vi "Picolog Close Device.vi"(8 "Error In":errorcluster, 11 "Instrument Handle":i16=1) -> (0 "Error Out":errorcluster)   [LabVIEW 2017]
uses:
  usbtc08.dll
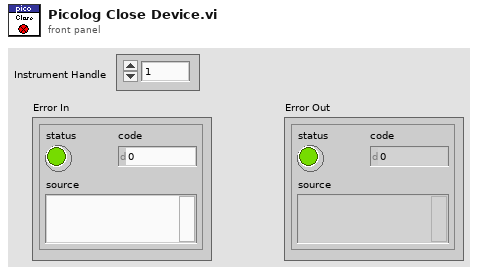
[diagram p1: front panel]
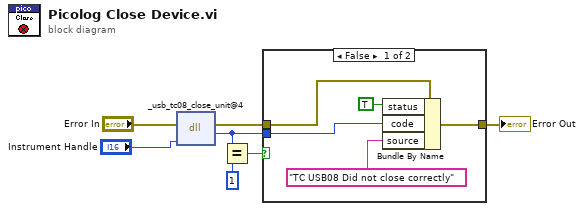
[diagram p0: block diagram]
diagram:
  n1 = dll-call lib="usbtc08.dll" fn="_usb_tc08_close_unit@4" label="Close unit"(error in="Error In", "handle"="Instrument Handle") -> (error out=w5:errorcluster, "return type"=w3:i16)  [unwired: 3 in, 1 out]
  n2 = Equal?(x=w3, y=i16 1) -> (x = y?=w1:bool)
  n3 = case shown="False" w1 {
    tunnel: [w8 w13] -> w4
    tunnel: w5 -> [w12 w13]
    tunnel: w3 -> [w10 _]
    frame False {
      n4 = Bundle By Name(cluster=w12, "status"=TRUE, "code"=w10, "source"="TC USB08 Did not close correctly") -> (w8:errorcluster)
    }
    frame True {
    }
  }
  "Error Out" <- w4
